vi "initialise.vi"(8 "error in (no error)":errorcluster, 11 "DL090324Microscope in":refnum<class "InstrumentDL090324.lvclass">) -> (0 "error out":errorcluster, 3 "DL090324Microscope out":refnum<class "InstrumentDL090324.lvclass">)   [LabVIEW 2010, in "InstrumentDL090324.lvclass"]
uses:
  InstrumentDL090324.lvclass
  GenericInstrument/GenericInstrument/GenericInstrument.lvclass
  InstrumentDL090324.lvclass/InstrumentDL090324.ctl
  Detector/GenericDetector/GenericDetector/GenericDetector.lvclass
  LightSource/GenericLightSource/GenericLightSource/GenericLightSource.lvclass
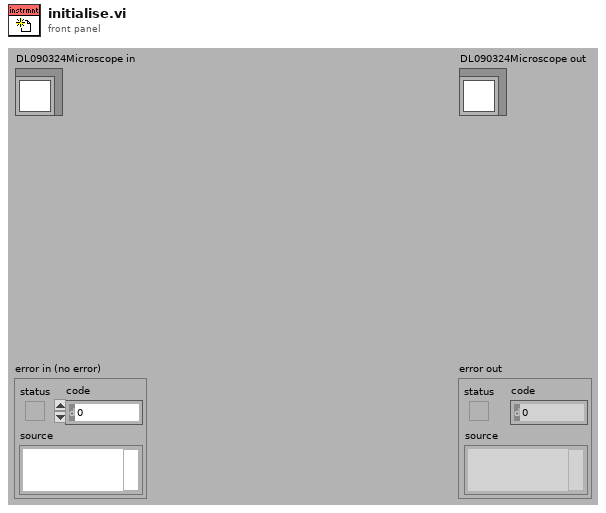
[diagram p1: front panel]
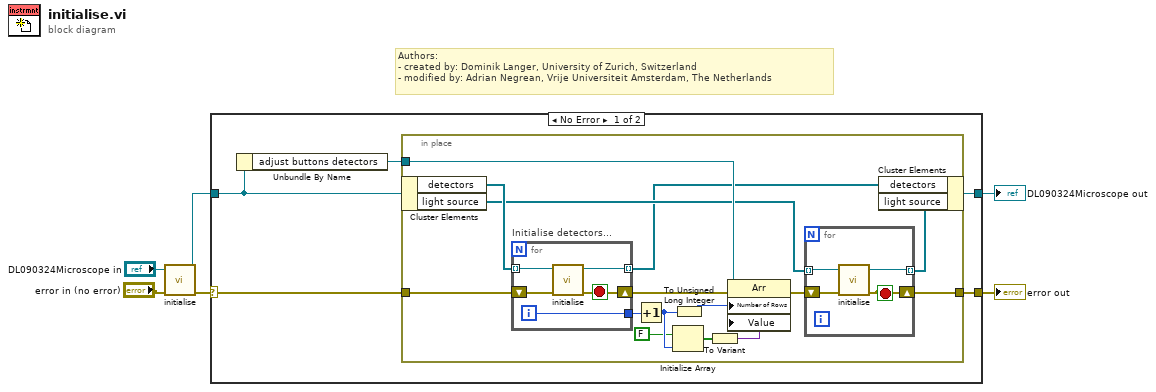
[diagram p0: block diagram]
diagram:
  # "Authors: \n- created by: Dominik Langer, University of Zurich, Switzerland\n- modified by: Adrian Negrean, Vrije Universiteit Amsterdam, The Netherlands"
  n1 = call-parent "initialise.vi"("error in (no error)"="error in (no error)", "GenericPlugin in"="DL090324Microscope in") -> ("error out"=w3:errorcluster, "GenericPlugin out"=w1:refnum<class "InstrumentDL090324.lvclass">)  [unwired: 8 out]
  n2 = case shown="No Error" w3 {
    selector: w3 -> [w10 w37]
    tunnel: [w9 w37] -> w6
    tunnel: [w7 w36] -> w5
    tunnel: w1 -> [w8 w36]
    frame No Error {
      n3 = Unbundle By Name(w8) -> ("adjust buttons detectors"=w11:refnum<vi>)
      n4 = in-place {
        in-place-border: w11 -> [w26]
        in-place-border: w10 -> [w20]
        in-place-border: [w12] -> w9
        n5 = in-place-cluster #1(w8) -> ("detectors"=w17:refnum<class "GenericDetector.lvclass">[], "light source"=w16:refnum<class "GenericLightSource.lvclass">[])
        n6 = for "Initialise detectors..." {
          shift-right: [w31] -> w19
          shift-left: w20 -> [w35]
          tunnel: w17 -> [w34] mode=indexing
          tunnel: [w33] -> w15 mode=indexing
          tunnel: [w32] -> w18
          i -> [w32]
          stop <- w31 stop-if-true
          n7 = call-dynamic "initialise.vi"("error in (no error)"=w35, "GenericPlugin in"=w34) -> ("error out"=w31:errorcluster, "GenericPlugin out"=w33:refnum<class "GenericDetector.lvclass">)  [unwired: 8 out]
        }
        n8 = Increment(x=w18) -> (x+1=w24:i32)
        n9 = Initialize Array(FALSE, w24) -> (w22:bool[])
        n10 = To Unsigned Long Integer(number=w24) -> (unsigned 32bit integer=w25:u32)
        n11 = To Variant(anything=w22) -> (Variant=w21:variant)
        n12 = property class="Arr"(reference=w26, error in=w19, "Number of Rows"=w25, "Value"=w21) -> (error out=w13:errorcluster)  [unwired: 1 out]
        n13 = for {
          tunnel: w16 -> [w29] mode=indexing
          tunnel: [w28] -> w14 mode=indexing
          shift-right: [w27] -> w12
          shift-left: w13 -> [w30]
          stop <- w27 stop-if-true
          n14 = call-dynamic "initialise.vi"("error in (no error)"=w30, "GenericPlugin in"=w29) -> ("error out"=w27:errorcluster, "GenericPlugin out"=w28:refnum<class "GenericLightSource.lvclass">)  [unwired: 8 out]
        }
        n15 = in-place-cluster #1("detectors"=w15, "light source"=w14) -> (w7:refnum<class "InstrumentDL090324.lvclass">)
      }
    }
    frame Error {
    }
  }
  "error out" <- w6
  "DL090324Microscope out" <- w5
